vi "AIT 1553 - Parse BC Sysdef Tree Messages.vi"(8 "error in":errorcluster, 9 "BC Messages In":T2[](array[typedef]), 10 "Section Ptr":T1 format="%.0x") -> (0 "error out":errorcluster, 1 "BC Messages Out":T2[](array[typedef]))   [LabVIEW 2013]
uses:
  <vilib>/NI Veristand/Custom Device API/Custom Device Item Ref.ctl
  Controls/1553_BC_Message.ctl
  Controls/1553 Param.ctl
  Controls and Global/Global.vi
  <vilib>/NI Veristand/Custom Device Tools/Custom Device Utility Library/NI VeriStand - Search for Item by Name.vi
  <vilib>/NI Veristand/Custom Device API/Get Item Property (I32).vi
  <vilib>/NI Veristand/Custom Device API/Get Item Property (Double).vi
  <vilib>/NI Veristand/Custom Device API/Get Item Property (Boolean).vi
  <vilib>/NI Veristand/Custom Device API/Custom Device API.lvlib
  AIT 1553 Custom Device.lvlib
  <vilib>/NI Veristand/Custom Device Tools/Custom Device Utility Library/Custom Device Utility Library.lvlib
panel:
  out "Found":bool[](array[boolean])
  out "Property Names":string[][][](array[string])
  out "Channel Refs":T1[][](array[typedef]) format="%.0x"
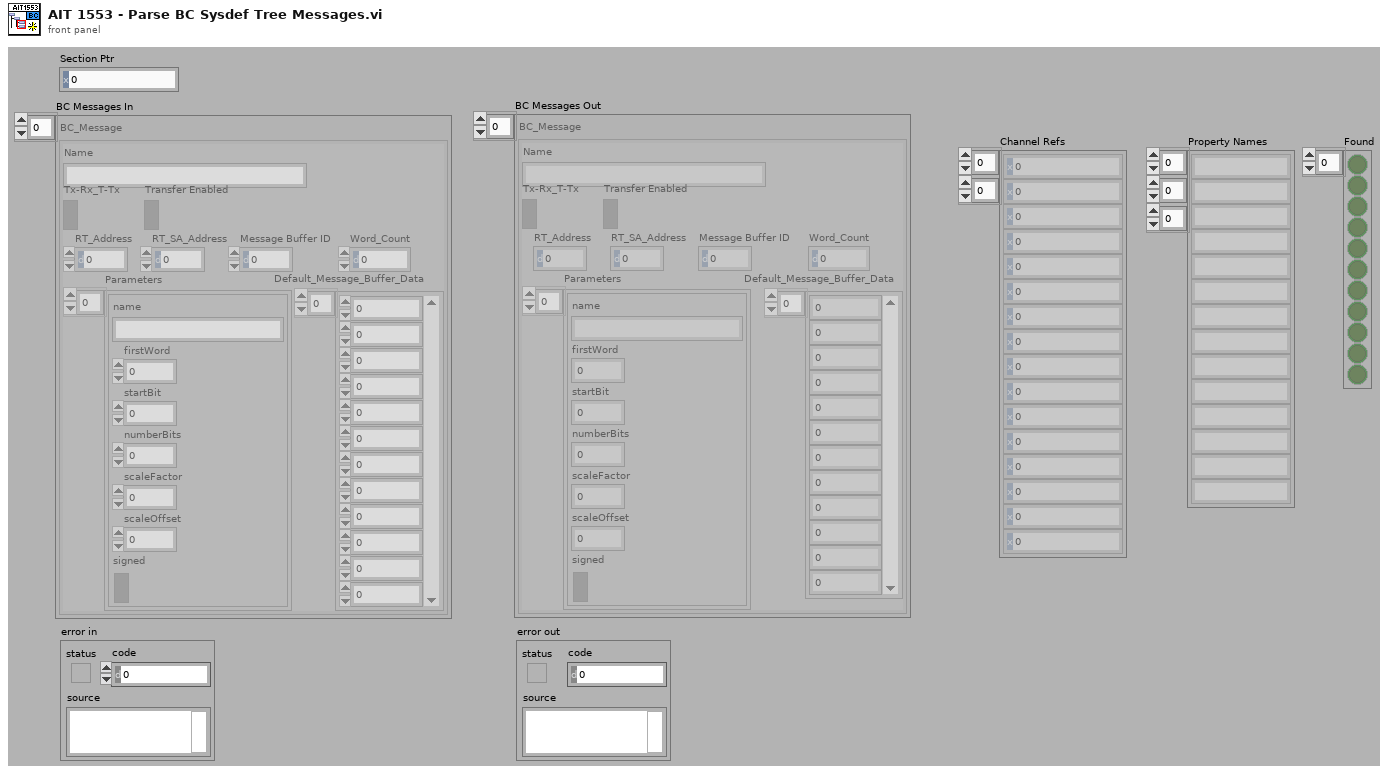
[diagram p1: front panel]
types:
  T1 = typedef "Custom Device API.lvlib/Custom Device Item Ref.ctl" = u64
  T2 = typedef "AIT 1553 Custom Device.lvlib/1553_BC_Message.ctl" = cluster{"Name":string, "Tx-Rx_T-Tx":bool, "RT_Address":u8, "RT_SA_Address":u8, "Parameters":T3[], "Transfer Enabled":bool, "Message Buffer ID":u16, "Default_Message_Buffer_Data":u16[], "Word_Count":u8}
  T3 = typedef "AIT 1553 Custom Device.lvlib/1553 Param.ctl" = cluster{"name":string, "firstWord":i32, "startBit":i32, "numberBits":i32, "scaleFactor":dbl, "scaleOffset":dbl, "signed":bool}
  T4 = enum32{"Invalid", "Standard", "Closed", "Hidden", "Minimized", "Maximized"}
  T5 = typedef "Custom Device API.lvlib/Custom Device Item Info.ctl" = cluster{"Name":string, "Is Channel":bool, "GUID":string, "Is Waveform":bool}
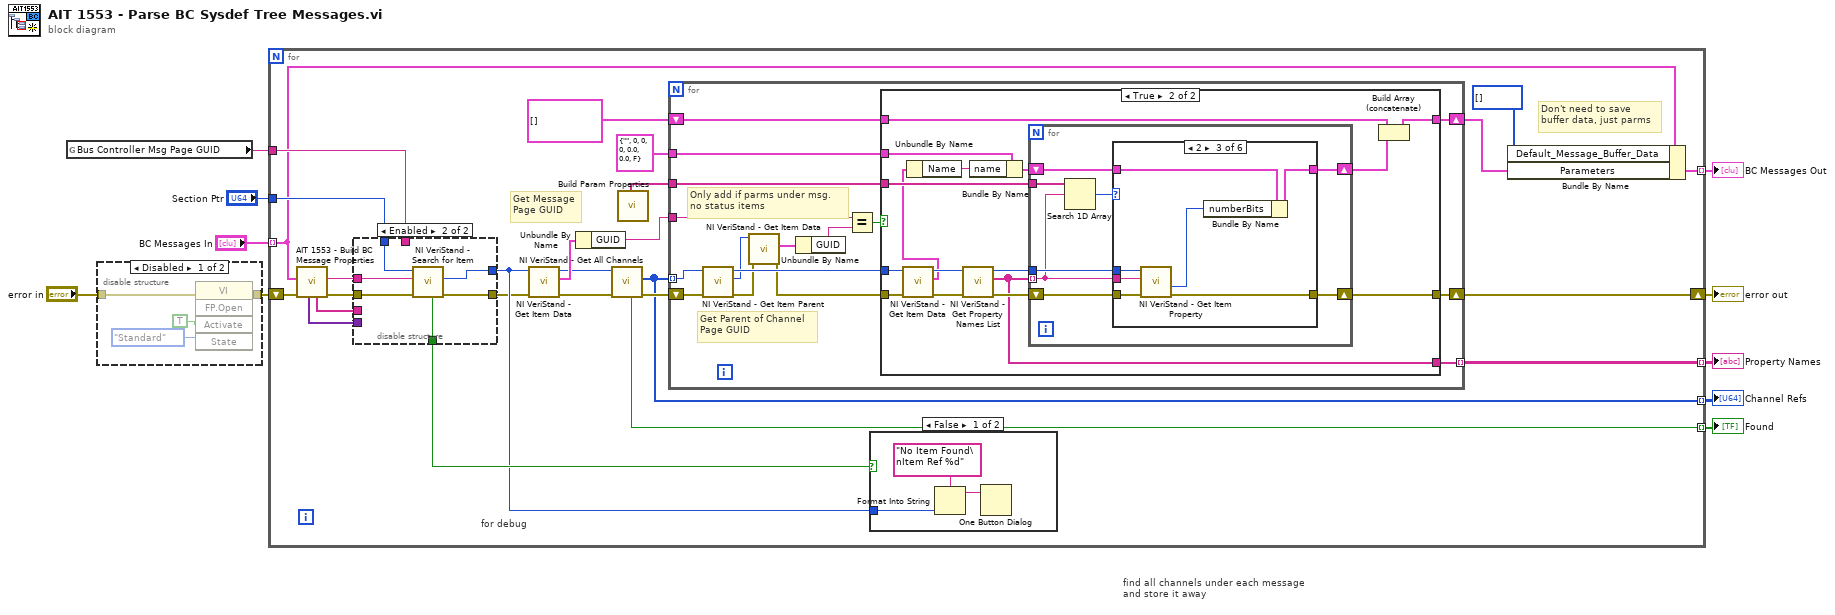
[diagram p0: block diagram]
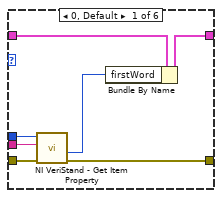
[diagram p5: hidden frame]
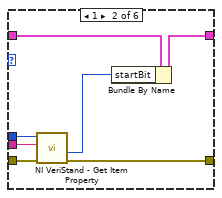
[diagram p6: hidden frame]
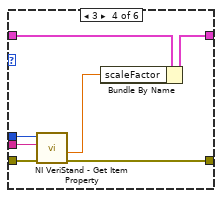
[diagram p7: hidden frame]
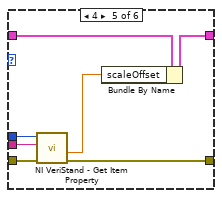
[diagram p8: hidden frame]
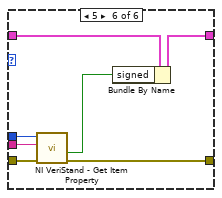
[diagram p9: hidden frame]
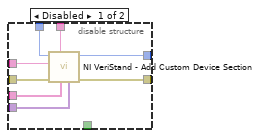
[diagram p10: hidden frame]
diagram:
  # "find all channels under each message\nand store it away"
  n1 = global read "Global.vi" "Bus Controller Msg Page GUID"() -> (w8:string)
  n2 = disable-structure shown="Disabled" {
    disable-tunnel: "error in" -> [w12 w15]
    disable-tunnel: [w11 w15] -> w4
    frame Disabled {
      n3 = invoke class="VI" method="FP.Open"(error in=w12, "Activate"=TRUE ("Activate?"), "State"=T4."Standard") -> (error out=w11:errorcluster)  [unwired: 2 in, 4 out]
    }
    frame Enabled {
    }
  }
  n4 = for {
    shift-right: [w16] -> w10
    shift-left: w4 -> [w37]
    tunnel: "Section Ptr" -> [w35]
    tunnel: "BC Messages In" -> [w32] mode=indexing
    tunnel: w8 -> [w36]
    tunnel: [w31] -> w6 mode=indexing
    tunnel: [w29] -> w3 mode=indexing
    tunnel: [w28] -> w2 mode=indexing
    tunnel: [w27] -> w1 mode=indexing
    # "Get Message\nPage GUID"
    # "Don't need to save\nbuffer data, just parms"
    # "for debug"
    n5 = call "AIT 1553 - Build BC Message Properties.vi"("error in (no error)"=w37, "BC_Message"=w32) -> ("error out"=w39:errorcluster, "name"=w38:string, "Prop Names"=w40:string[], "Prop Values"=w41:variant[])  [unwired: 5 in, 1 out]
    n6 = disable-structure shown="Enabled" {
      disable-tunnel: w41 -> [w136 _]
      disable-tunnel: w40 -> [w135 _]
      disable-tunnel: w39 -> [w134 w141]
      disable-tunnel: w38 -> [w133 w142]
      disable-tunnel: w36 -> [w132 _]
      disable-tunnel: w35 -> [w131 w140]
      disable-tunnel: [w130 w137] -> w18
      disable-tunnel: [w129 w139] -> w24
      disable-tunnel: [_ w138] -> w30
      frame Disabled {
        n7 = call <vilib>:"NI VeriStand - Add Custom Device Section.vi"("Property Values"=w136, "Property names"=w135, "GUID (Default Section)"=w132, "error in (no error)"=w134, "Section Name"=w133, "Parent Ref in"=w131) -> ("error out"=w130:errorcluster, "Section Ptr"=w129:T1)  [unwired: 2 in, 2 out]
      }
      frame Enabled {
        n8 = call-poly <vilib>:"NI VeriStand - Search for Item.vi"("error in"=w141, "Item Name"=w142, "Section Ref in"=w140) -> ("error out"=w137:errorcluster, "Item Ref"=w139:T1, "Found"=w138:bool)  [unwired: 5 in, 1 out]
      }
    }
    n9 = call <vilib>:"NI VeriStand - Get Item Data.vi"("error in (no error)"=w18, "Item Ref in"=w24) -> ("error out"=w17:errorcluster, "Item Info"=w23:T5, "Item Ref out"=w19:T1)  [unwired: 6 in, 1 out]
    n10 = Unbundle By Name(w23) -> ("GUID"=w22:string)
    n11 = call <vilib>:"NI VeriStand - Get All Channels.vi"("error in"=w17, "Section Ref in"=w19) -> ("error out"=w34:errorcluster, "Channel Refs"=w28:T1[], "Found"=w29:bool)  [unwired: 6 in, 1 out]
    n12 = call "Build Param Properties.vi"() -> ("Prop Names"=w33:string[])  [unwired: 11 in, 8 out]
    n13 = for {
      tunnel: w28 -> [w55] mode=indexing
      tunnel: w33 -> [w60]
      tunnel: [w57] -> w27 mode=indexing
      tunnel: T3 {"name"="", "firstWord"=0, "startBit"=0, "numberBits"=0, "scaleFactor"=0.0, "scaleOffset"=0.0, "signed"=FALSE} ("1553 Parameter") -> [w58]
      tunnel: w22 -> [w48]
      shift-right: [w45] -> w20
      shift-left: T3[] [] -> [w46]
      shift-right: [w59] -> w16
      shift-left: w34 -> [w56]
      # "Only add if parms under msg.\nno status items"
      # "Get Parent of Channel\nPage GUID"
      n14 = call <vilib>:"NI VeriStand - Get Item Parent.vi"("error in (no error)"=w56, "Item Ref in"=w55) -> ("error out"=w53:errorcluster, "Parent Ref"=w51:T1, "Item Ref out"=w54:T1)  [unwired: 6 in, 1 out]
      n15 = call <vilib>:"NI VeriStand - Get Item Data.vi"("error in (no error)"=w53, "Item Ref in"=w51) -> ("error out"=w52:errorcluster, "Item Info"=w50:T5)  [unwired: 6 in, 2 out]
      n16 = Unbundle By Name(w50) -> ("GUID"=w49:string)
      n17 = Equal?(x=w48, y=w49) -> (x = y?=w47:bool)
      n18 = case shown="True" w47 {
        tunnel: w60 -> [_ w77]
        tunnel: [w61 w63] -> w59
        tunnel: w58 -> [_ w73]
        tunnel: [_ w69] -> w57
        tunnel: w54 -> [_ w68]
        tunnel: w52 -> [w61 w67]
        tunnel: w46 -> [w62 w66]
        tunnel: [w62 w64] -> w45
        frame False {
        }
        frame True {
          n19 = call <vilib>:"NI VeriStand - Get Item Data.vi"("error in (no error)"=w67, "Item Ref in"=w68) -> ("error out"=w75:errorcluster, "Item Info"=w70:T5, "Item Ref out"=w74:T1)  [unwired: 6 in, 1 out]
          n20 = Unbundle By Name(w70) -> ("Name"=w71:string)
          n21 = call <vilib>:"NI VeriStand - Get Property Names List.vi"("error in (no error)"=w75, "Item Ref in"=w74) -> ("error out"=w78:errorcluster, "Property Names"=w69:string[], "Item Ref out"=w76:T1)  [unwired: 7 in]
          n22 = Bundle By Name(cluster=w73, "name"=w71) -> (w72:T3)
          n23 = for {
            tunnel: w69 -> [w81] mode=indexing
            tunnel: w77 -> [w86]
            shift-right: [w80] -> w65
            shift-left: w72 -> [w84]
            tunnel: w76 -> [w82]
            shift-right: [w79] -> w63
            shift-left: w78 -> [w83]
            n24 = Search 1D Array(1D array=w86, element=w81) -> (index of element=w85:i32)  [unwired: 1 in]
            n25 = case shown="2" w85 {
              tunnel: w84 -> [w93 w100 w107 w114 w121 w128]
              tunnel: w83 -> [w92 w99 w106 w113 w120 w127]
              tunnel: w82 -> [w91 w98 w105 w112 w119 w126]
              tunnel: w81 -> [w90 w97 w104 w111 w118 w125]
              tunnel: [w88 w95 w102 w109 w116 w123] -> w80
              tunnel: [w87 w94 w101 w108 w115 w122] -> w79
              frame 0, Default {
                n26 = call-poly <vilib>:"NI VeriStand - Get Item Property.vi"("error in (no error)"=w92, "Property Name"=w90, "Item Ref in"=w91) -> ("error out"=w87:errorcluster, "Value"=w89:i32)  [unwired: 5 in, 2 out]
                n27 = Bundle By Name(cluster=w93, "firstWord"=w89) -> (w88:T3)
              }
              frame 1 {
                n28 = call-poly <vilib>:"NI VeriStand - Get Item Property.vi"("error in (no error)"=w99, "Property Name"=w97, "Item Ref in"=w98) -> ("error out"=w94:errorcluster, "Value"=w96:i32)  [unwired: 5 in, 2 out]
                n29 = Bundle By Name(cluster=w100, "startBit"=w96) -> (w95:T3)
              }
              frame 2 {
                n30 = call-poly <vilib>:"NI VeriStand - Get Item Property.vi"("error in (no error)"=w106, "Property Name"=w104, "Item Ref in"=w105) -> ("error out"=w101:errorcluster, "Value"=w103:i32)  [unwired: 5 in, 2 out]
                n31 = Bundle By Name(cluster=w107, "numberBits"=w103) -> (w102:T3)
              }
              frame 3 {
                n32 = call-poly <vilib>:"NI VeriStand - Get Item Property.vi"("error in (no error)"=w113, "Property Name"=w111, "Item Ref in"=w112) -> ("error out"=w108:errorcluster, "Value"=w110:dbl)  [unwired: 5 in, 2 out]
                n33 = Bundle By Name(cluster=w114, "scaleFactor"=w110) -> (w109:T3)
              }
              frame 4 {
                n34 = call-poly <vilib>:"NI VeriStand - Get Item Property.vi"("error in (no error)"=w120, "Property Name"=w118, "Item Ref in"=w119) -> ("error out"=w115:errorcluster, "Value"=w117:dbl)  [unwired: 5 in, 2 out]
                n35 = Bundle By Name(cluster=w121, "scaleOffset"=w117) -> (w116:T3)
              }
              frame 5 {
                n36 = call-poly <vilib>:"NI VeriStand - Get Item Property.vi"("error in (no error)"=w127, "Property Name"=w125, "Item Ref in"=w126) -> ("error out"=w122:errorcluster, "Value"=w124:bool)  [unwired: 5 in, 2 out]
                n37 = Bundle By Name(cluster=w128, "signed"=w124) -> (w123:T3)
              }
            }
          }
          n38 = Build Array (concatenate)(w66, w65) -> (w64:T3[])
        }
      }
    }
    n39 = case shown="False" w30 {
      tunnel: w24 -> [w44 _]
      frame False {
        n40 = Format Into String(format string="No Item Found\nItem Ref %d" ("message"), w44) -> (resulting string=w43:string)  [unwired: 2 in, 1 out]
        n41 = One Button Dialog(message=w43) -> ()  [unwired: 1 in, 1 out]
      }
      frame True {
      }
    }
    n42 = Bundle By Name(cluster=w32, "Default_Message_Buffer_Data"=u16[] [], "Parameters"=w20) -> (w31:T2)
  }
  "error out" <- w10
  "BC Messages Out" <- w6
  "Found" <- w3
  "Channel Refs" <- w2
  "Property Names" <- w1
